vi "Poll Turbo Valve Control.vi"(8 "error in (no error)":errorcluster, 11 "Turbo in":refnum<class "Turbo.lvclass">) -> ()   [LabVIEW 2015, in "cRIO-Carbondioxide.lvlib" / "CO2-Actor.lvlib" / "Turbo.lvclass"]
uses:
  Turbo.lvclass
  Turbo.lvclass/Turbo.ctl
  <vilib>/ActorFramework/Actor/Actor.lvclass/Actor.ctl
  <vilib>/ActorFramework/Message Enqueuer/Message Enqueuer.lvclass/Message Enqueuer.ctl
  Turbo Messages/Set Turbo Valve Msg/Set Turbo Valve Msg.lvclass/Set Turbo Valve Msg.ctl
  <vilib>/ActorFramework/Actor/Read Self Enqueuer.vi
  <vilib>/ActorFramework/Message Enqueuer/Enqueue.vi
  <vilib>/ActorFramework/Message Enqueuer/Init from Existing Queue.vi
  <vilib>/ActorFramework/Message Priority Queue/Priority Enqueue.vi
  <vilib>/ActorFramework/Actor/Actor.lvclass
  <vilib>/ActorFramework/Message Enqueuer/Message Enqueuer.lvclass
  Turbo Messages/Set Turbo Valve Msg/Set Turbo Valve Msg.lvclass
  CO2 Actor/CO2 Actor.lvclass
  cRIO-CO2/cRIO-CO2.lvclass
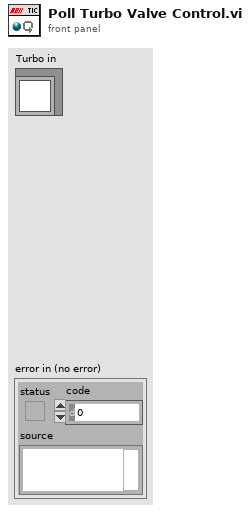
[diagram p1: front panel]
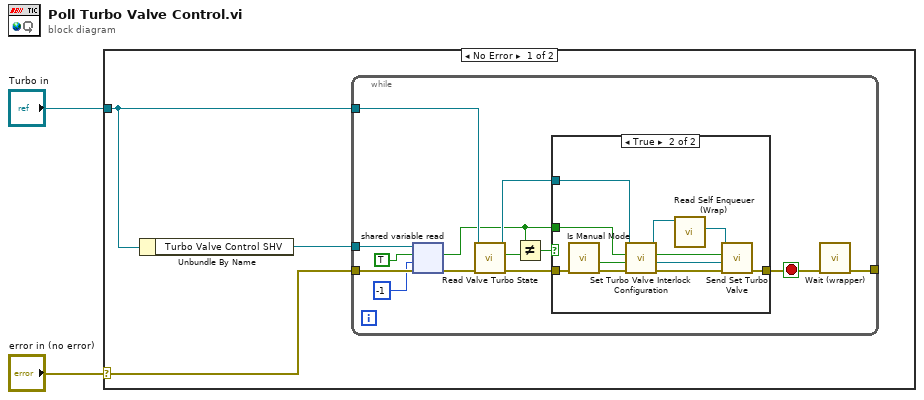
[diagram p0: block diagram]
diagram:
  n1 = case shown="No Error" "error in (no error)" {
    selector: "error in (no error)" -> [w4 _]
    tunnel: "Turbo in" -> [w3 _]
    frame No Error {
      n2 = Unbundle By Name(w3) -> ("Turbo Valve Control SHV"=w5:refnum<k21>)
      n3 = while {
        tunnel: w5 -> [w18]
        tunnel: w4 -> [w17]
        tunnel: w3 -> [w12]
        tunnel: [w6] -> _
        stop <- w7 stop-if-true
        n4 = shared-variable-read(w18, w17, TRUE, -1 ("timeout ms")) -> (w14:errorcluster, w9:bool)  [unwired: 3 out]
        n5 = call "Read Valve Turbo State.vi"("error in (no error)"=w14, "Turbo in"=w12) -> ("error out"=w13:errorcluster, "Open?"=w10:bool, "Turbo out"=w11:refnum<class "Turbo.lvclass">)  [unwired: 6 in, 1 out]
        n6 = Not Equal?(x=w9, y=w10) -> (x != y?=w8:bool)
        n7 = case shown="True" w8 {
          tunnel: [w19 w30] -> w7
          tunnel: w9 -> [_ w20]
          tunnel: w13 -> [w19 w22]
          tunnel: w11 -> [_ w21]
          frame False {
          }
          frame True {
            n8 = call "Is Manual Mode.vi"("error in (no error)"=w22) -> ("error out"=w29:errorcluster, "Manual Mode?"=w25:bool)  [unwired: 9 in]
            n9 = call "Set Turbo Valve Interlock Configuration.vi"("error in (no error)"=w29, "Manual Mode (False)"=w25, "Open? (False)"=w20, "Turbo in"=w21) -> ("error out"=w28:errorcluster, "Interlock Chain"=w24:refnum<class "Interlock Chain.lvclass">, "Open? (False) 2"=w23:bool, "Turbo out"=w26:refnum<class "Turbo.lvclass">)  [unwired: 4 in]
            n10 = call "Read Self Enqueuer (Wrap).vi"("CO2 Actor in"=w26) -> ("Actor Framework:Message Enqueuer"=w27:refnum<class "Message Enqueuer.lvclass">)  [unwired: 9 in, 1 out]
            n11 = call "Send Set Turbo Valve.vi"("error in (no error)"=w28, "Interlock Chain.lvclass"=w24, "Open? (False)"=w23, "Message Enqueuer"=w27) -> ("error out"=w30:errorcluster)  [unwired: 6 in, 1 out]
          }
        }
        n12 = call "Wait (wrapper).vi"("error in (no error)"=w7) -> ("error out"=w6:errorcluster)  [unwired: 10 in]
      }
    }
    frame Error {
    }
  }
